vi "Current VI Path.vi"(1 "file name":string="open.txt") -> (0 "Path for file":path)   [LabVIEW 2014]
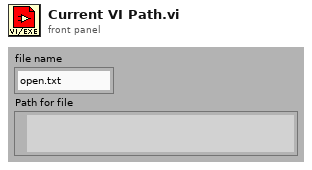
[diagram p1: front panel]
types:
  T1 = enum32{"invalid OS target", "Mac OS", "Windows 3.1", "Windows 95/NT", "Solaris 1", "Solaris 2", "HP-UX", "PowerMAX", "Linux", "Irix", "Rhapsody", "BeOS", "AIX", "OSF1", "VxWorks", "PharLap", "Carbon", "RTX", "Windows x64", "Linux x64", "Mac OS X x64"}
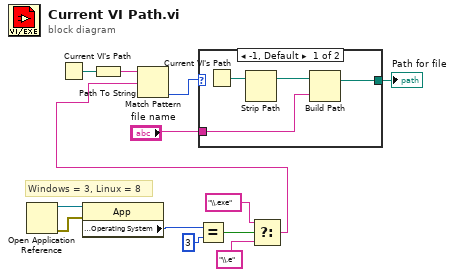
[diagram p0: block diagram]
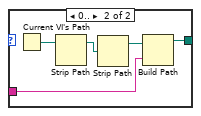
[diagram p2: hidden frame]
diagram:
  # "Windows = 3, Linux = 8"
  n1 = Open Application Reference() -> (0:w4:errorcluster, 3:w5:refnum<vi>)  [unwired: 4 in]
  n2 = Current VI's Path() -> (path=w13:path)
  n3 = property class="App"(reference=w5, error in=w4) -> ("Application:Target:Operating System"=w3:T1)  [unwired: 2 out]
  n4 = Path To String(path=w13) -> (string=w12:string)
  n5 = Equal?(x=w3, y=3) -> (x = y?=w7:bool)
  n6 = Select(t="\\.exe" ("file name"), s=w7, f="\\.e" ("file name")) -> (s? t:f=w1:string)
  n7 = Match Pattern(string=w12, regular expression=w1) -> (offset past match=w11:i32)  [unwired: 1 in, 3 out]
  n8 = case shown="-1, Default" w11 {
    tunnel: [w15 w21] -> w10
    tunnel: "file name" -> [w14 w20]
    frame -1, Default {
      n9 = Current VI's Path() -> (path=w17:path)
      n10 = Strip Path(path=w17) -> (stripped path=w16:path)  [unwired: 1 out]
      n11 = Build Path(base path=w16, name or relative path=w14) -> (appended path=w15:path)
    }
    frame 0.. {
      n12 = Current VI's Path() -> (path=w22:path)
      n13 = Strip Path(path=w22) -> (stripped path=w19:path)  [unwired: 1 out]
      n14 = Strip Path(path=w19) -> (stripped path=w18:path)  [unwired: 1 out]
      n15 = Build Path(base path=w18, name or relative path=w20) -> (appended path=w21:path)
    }
  }
  "Path for file" <- w10
